vi "hardware_close_hardware.vi"(8 "error in (no error)":errorcluster, 11 "lightfield_class in":refnum<class "lightfield_class.lvclass">) -> (0 "error out":errorcluster, 3 "lightfield_class out":refnum<class "lightfield_class.lvclass">)   [LabVIEW 2015, in "lightfield_class.lvclass"]
uses:
  lightfield_class.lvclass
  lightfield_class.lvclass/lightfield_class.ctl
  lightfield-automation-labview/LightField Automation.lvclass
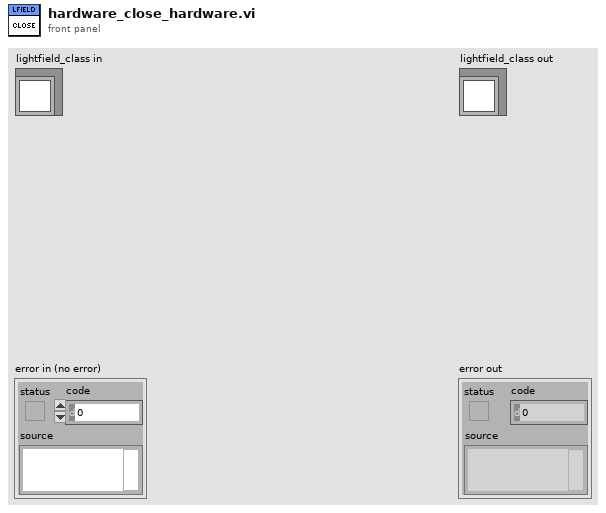
[diagram p1: front panel]
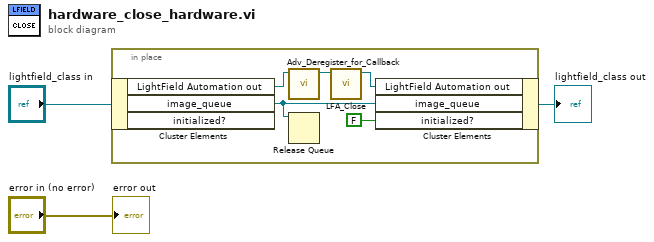
[diagram p0: block diagram]
diagram:
  n1 = in-place {
    n2 = in-place-cluster #1("lightfield_class in") -> ("LightField Automation out"=w7:refnum<class "LightField Automation.lvclass">, "image_queue"=w5:refnum<queue>)  [unwired: 1 out]
    n3 = call "Adv_Deregister_for_Callback.vi"("LightField Automation in"=w7) -> ("LightField Automation out"=w6:refnum<class "LightField Automation.lvclass">)  [unwired: 9 in, 1 out]
    n4 = Release Queue(queue=w5) -> ()  [unwired: 2 in, 3 out]
    n5 = call "LFA_Close.vi"("LightField Automation in"=w6) -> ("LightField Automation out"=w8:refnum<class "LightField Automation.lvclass">)  [unwired: 9 in, 1 out]
    n6 = in-place-cluster #1("LightField Automation out"=w8, "image_queue"=w5, "initialized?"=FALSE) -> (→"lightfield_class out":refnum<class "lightfield_class.lvclass">)
  }
  "error out" <- "error in (no error)"
